vi "FPGA Main (3 Motor).vi"() -> ()   [LabVIEW 2013]
uses:
  Sub VIs/Utilities/Start Boolean.ctl
  <vilib>/Platform/TimedLoop/XDataNode/timing_clust.ctl
  <vilib>/Platform/TimedLoop/XDataNode/nitl_modes.ctl
  <vilib>/Platform/TimedLoop/XDataNode/wakeup.ctl
  <vilib>/rvi/Emulation/niFpgaSctlEmulationGetInTimedLoop.vi
  <vilib>/rvi/Emulation/niFpgaEmulationReportErrorSimple.vi
  <vilib>/rvi/Emulation/niFpgaGetClockAttributes.vi
  <vilib>/rvi/Emulation/niFpgaCriticalErrorInLSC.vi
  <vilib>/rvi/eio/common/nirviEmuTemplateMethod_errors.vi
  <vilib>/rvi/eio/common/nirviEmuTemplatePropertyGet_noerrors.vi
  <vilib>/rvi/interface/RandomDataEmulation/nirviRandomDataFPGAFIFO.vi
  <vilib>/rvi/interface/RandomDataEmulation/niFpgaRandomDataHandleErrors.vi
  <vilib>/Platform/TimedLoop/XDataNode/XDataNode.xnode
  <vilib>/eio/EIONode/EIONode.xnode
  <vilib>/eio/EIOPropertyNode/EIOPropertyNode.xnode
  <vilib>/rvi/DataTransferAndStorage/Container/XNode/niFpgaContainer.xnode
  <vilib>/rvi/interface/RandomDataEmulation/nirviRandomDataFpgaReadWriteTemplate.vi
  <vilib>/Platform/TimedLoop/XDataNode/XDNodeRunTimeDep.lvlib
  <vilib>/rvi/eio/common/nirviEmuTemplatePropertyGet_errors.vi
  <vilib>/rvi/eio/common/nirviEmuTemplatePropertySet_errors.vi
  <vilib>/rvi/eio/common/nirviEmuTemplatePropertySet_noerrors.vi
panel:
  out "Diff_EncC0":u32
  out "Diff_EncB":u32
  out "Diff_EncA":u32
  in  "ABS Enc Channel":u8=255
  in  "Recieved (ticks)":u32=1389
  out "SYS.ACC_SCALE.RDY":bool
  out "ACC.SCALE.WGHT":u16
  out "AO.A_0.WGHT":u32
  out "AO.A_1.WGHT":u32
  out "AO.C_0.WGHT":u32
  out "AO.C_1.WGHT":u32
  out "AO.AudioOut_L.WGHT":u32
  out "AO.AudioOut_R.WGHT":u32
  out "AO.A_0.OFST":u32
  out "AO.C_0.OFST":u32
  out "AO.C_1.OFST":u32
  out "AO.AudioOut_L.OFST":u32
  out "AO.AudioOut_R.OFST":u32
  out "AO.A_1.OFST":u32
  out "SYS.AO_SCALE.RDY":bool
  out "AO.B_0.WGHT":u32
  out "AO.B_1.WGHT":u32
  out "AO.B_0.OFST":u32
  out "AO.B_1.OFST":u32
  out "AI.A_0.WGHT":u32
  out "AI.A_1.WGHT":u32
  out "AI.A_2.WGHT":u32
  out "AI.A_3.WGHT":u32
  out "AI.B_0.WGHT":u32
  out "AI.B_2.WGHT":u32
  out "AI.B_3.WGHT":u32
  out "AI.C_0.WGHT":u32
  out "AI.C_1.WGHT":u32
  out "AI.AudioIn_L.WGHT":u32
  out "AI.AudioIn_R.WGHT":u32
  out "AI.A_0.OFST":u32
  out "AI.A_2.OFST":u32
  out "AI.A_3.OFST":u32
  out "AI.B_0.OFST":u32
  out "AI.B_1.OFST":u32
  out "AI.B_2.OFST":u32
  out "AI.B_3.OFST":u32
  out "AI.C_0.OFST":u32
  out "AI.C_1.OFST":u32
  out "AI.AudioIn_L.OFST":u32
  out "AI.AudioIn_R.OFST":u32
  out "AI.A_1.OFST":u32
  out "SYS.AI_SCALE.RDY":bool
  out "AI.B_1.WGHT":u32
  out "ACC.Z.VAL":u16
  out "SYS.ACC.RDY":bool
  out "ACC.Y.VAL":u16
  out "ACC.X.VAL":u16
  in  "DO.LED3:0":u8 format="%04b"
  out "DI.BTN":u8 format="%08b"
  in  "SYS.SELECTB":u8 format="%08b"
  in  "DIO.B_7:0.DIR":u8 format="%08b"
  in  "DIO.B_7:0.OUT":u8 format="%08b"
  in  "DIO.B_15:8.DIR":u8 format="%08b"
  in  "DIO.B_15:8.OUT":u8 format="%08b"
  out "DIO.B_7:0.IN":u8 format="%08b"
  out "DIO.B_15:8.IN":u8 format="%08b"
  in  "ENC.B.CNFG":u8 format="%08b"
  out "ENC.B.CNTR":u32
  out "ENC.B.STAT":u8 format="%08b"
  out "SYS.RDY":bool
  out "AI.A_0.VAL":u16
  out "AI.A_1.VAL":u16
  out "AI.A_2.VAL":u16
  out "AI.A_3.VAL":u16
  out "AI.B_0.VAL":u16
  out "AI.B_1.VAL":u16
  out "AI.B_2.VAL":u16
  out "AI.B_3.VAL":u16
  out "SYS.AI.RDY":bool
  out "AI.AudioIn_L.VAL":u16
  out "AI.AudioIn_R.VAL":u16
  out "AI.C_1.VAL":u16
  out "AI.C_0.VAL":u16
  in  "AO.A_0.VAL":u16
  in  "AO.A_1.VAL":u16
  in  "AO.B_0.VAL":u16
  in  "AO.B_1.VAL":u16
  in  "AO.AudioOut_L.VAL":u16
  in  "AO.AudioOut_R.VAL":u16
  in  "AO.SYS.GO":T1
  in  "AO.C_1.VAL":u16
  in  "AO.C_0.VAL":u16
  out "AO.SYS.STAT":bool
  in  "SYS.SELECTA":u8 format="%08b"
  in  "DIO.A_7:0.OUT":u8 format="%08b"
  in  "DIO.A_7:0.DIR":u8 format="%08b"
  out "DIO.A_7:0.IN":u8 format="%08b"
  in  "DIO.A_15:8.OUT":u8 format="%08b"
  in  "DIO.A_15:8.DIR":u8 format="%08b"
  out "DIO.A_15:8.IN":u8 format="%08b"
  in  "PWM.A_0.MAX":u16
  in  "PWM.A_0.CMP":u16
  in  "PWM.A_0.CNFG":u8 format="%08b"
  in  "PWM.A_0.CS":u8
  out "PWM.A_0.CNTR":u16
  in  "PWM.A_1.CMP":u16
  in  "PWM.A_1.MAX":u16
  out "PWM.A_1.CNTR":u16
  in  "PWM.A_1.CNFG":u8 format="%08b"
  in  "PWM.A_1.CS":u8
  in  "PWM.A_2.CMP":u16
  in  "PWM.A_2.MAX":u16
  out "PWM.A_2.CNTR":u16
  in  "PWM.A_2.CNFG":u8 format="%08b"
  in  "PWM.A_2.CS":u8
  in  "ENC.A.CNFG":u8 format="%08b"
  out "ENC.A.CNTR":u32
  out "ENC.A.STAT":u8 format="%08b"
  out "DIO.C_7:0.IN":u8 format="%08b"
  in  "DIO.C_7:0.DIR":u8 format="%08b"
  in  "DIO.C_7:0.OUT":u8 format="%08b"
  in  "ENC.C_0.CNFG":u8 format="%08b"
  out "ENC.C_0.CNTR":u32
  out "ENC.C_0.STAT":u8 format="%08b"
  in  "SYS.SELECTC":u8 format="%08b"
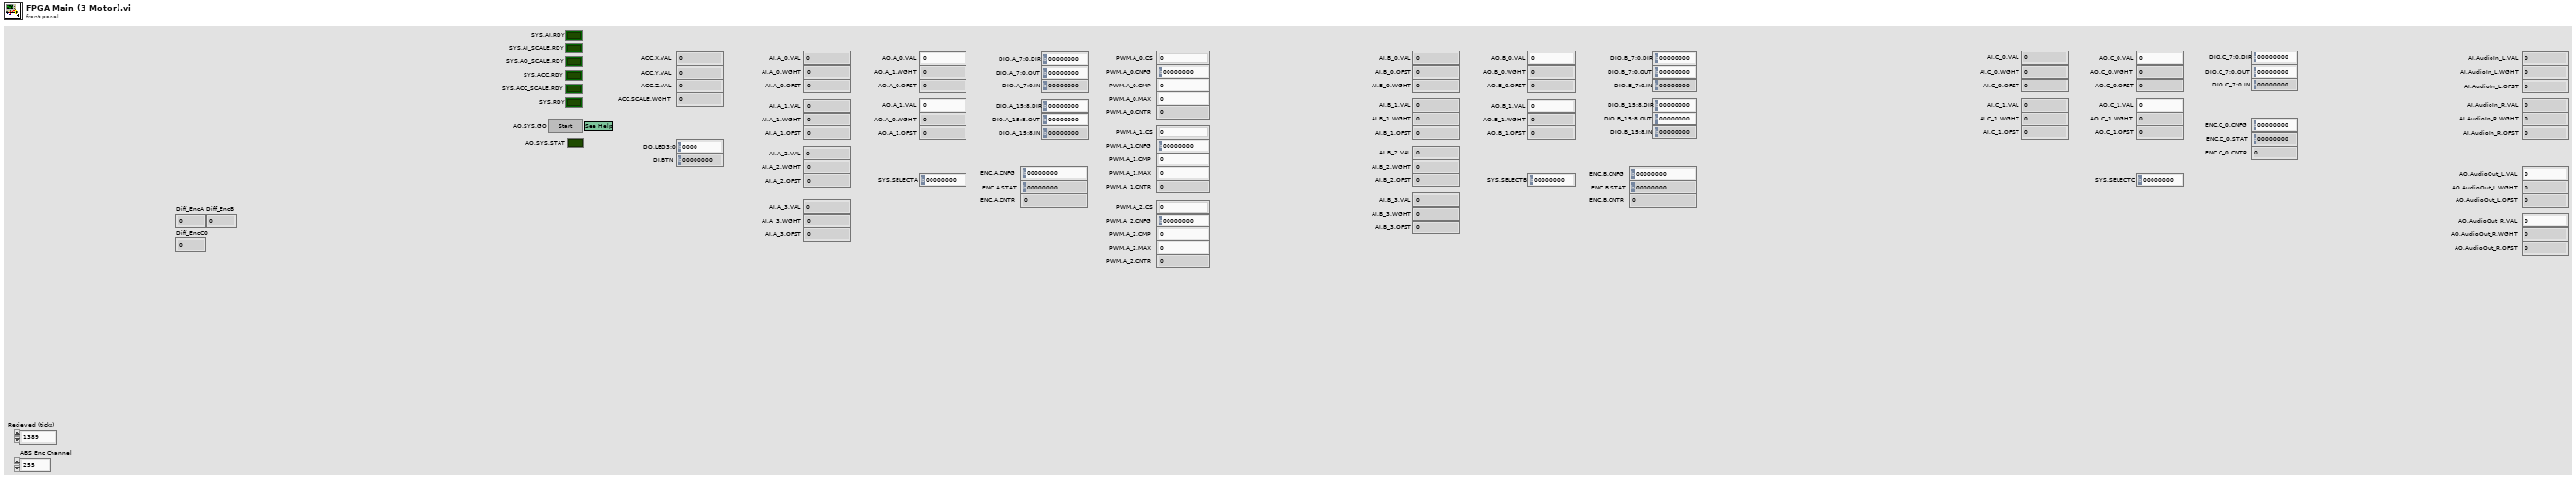
[diagram p1: front panel]
types:
  T1 = typedef "Start Boolean.ctl" = bool
  T2 = typedef "XDNodeRunTimeDep.lvlib/timing_clust.ctl" = cluster{"Expected End [f-1]":u64, "Actual End [f-1]":u64, "Finished Late? [f-1]":bool, "Expected End [i-1]":u64, "Actual End [i-1]":u64, "Finished Late? [i-1]":bool, "Expected Start [i]":u64, "Actual Start [i]":u64, "Expected Start [f]":u64, "Actual Start [f]":u64, "Source Name":string, "Structure Name":string, "Period":i64, "Deadline":i64, "Offset":i64, "Start":i64, "Priority":i32, "Timeout":i32, "Mode":T3, "Wakeup Reason":T4, "Error":errorcluster, "Source Type":string, "Secondary Source Type":string, "Global End Time":u64, "Global Start Time":u64, "Frame Duration":u64, "Iteration Duration":u64, "Assigned CPU":i32, "I/O Scan Engine Mode":u32}
  T3 = typedef "XDNodeRunTimeDep.lvlib/nitl_modes.ctl" = enum32{"No Change", "Process missed periods, maintain original phase", "Discard missed periods, maintain original phase", "Process missed periods, ignore original phase", "Discard missed periods, ignore original phase"}
  T4 = typedef "XDNodeRunTimeDep.lvlib/wakeup.ctl" = enum32{"Normal", "Aborted", "Asynchronous wakeup", "Timing source error", "Timed loop error", "Timeout"}
diagram:
  w1 = u32 0 ("ENC.B.CNTR")
  # "NOTE: The SYS.RDY boolean MUST exist and must become TRUE at some point otherwise the myRIO API will not function correctly."
  # "All DIO operations occur inside one single cycle timed loop (SCTL) since the IO is shared."
  # "The analog input scaling values are stored on the hardware. The RDY boolean should be checked before the values are used otherwise the analog input vlaues could be scaled incorrectly.\n\nAfter the first iteration of the while loop, all indicators have valid values."
  # "The analog output scaling values are stored on the hardware. The RDY boolean should be checked before the values are used otherwise the analog output vlaues could be scaled incorrectly.\n\nAfter the first iteration of the while loop, all indicators have valid values."
  # "The accelerometer nodes takes some time before the values can first be read (this is due to the time taken to read from the acceleromter). An iteration of the while loop will not complete until the accelerometer values have been read.\n\nAfter the first iteration of the while loop, all indicators have valid values."
  # "The onboard accelerometer has a range of +/- 8g which translates to 256 bits/g. The scaling weight is hardcoded in the FPGA to allow for future updates with minimal changes in the myRIO code. The RDY boolean should be checked before the values are used otherwise the analog output vlaues could be scaled incorrectly.\n\nAfter the first iteration of the while loop, all indicators have valid values."
  # "Onboard Accelerometer Scaling"
  # "Analog Output Scaling Constants"
  # "Analog Input Scaling Constants"
  # "Onboard Accelerometer"
  # "Onboard DIO"
  # "Connector B DIO"
  # "There is some delay between when the FPGA code starts and the analog inputs, accelerometer, and scaling values outputs are valid. If the host wants to ensure that there are valid values in theses registers it should wait for each subsystem to finish its initialization process. \n\nWhen all subsystems have finished initializinig, the SYS.RDY indicator will be true, which can be polled by the host to determine the status of the FPGA. Alternatively, the host can poll the individual SYS.xx.RDY indicators to determine the status of the individual subsystems.\n\nThis loop continues indefinitely, essentially making SYS.RDY a read-only register."
  # "The analog input nodes takes some time before the values can first be read (this is due to the time taken to setup the ADC and convert the first reading). An iteration of the while loop will not complete until all the analog input channels have been sampled.\n\nAfter the first iteration of the while loop, all indicators have valid values."
  # "Note: On some hardware a \"ghosting effect\" may occur on any unconnected AI channels. For example, if channel AI0 is connected and channels AI1 - AI7 are not connected the the value read at AI0 may be seen on indicators AI1 - AI7. This is common for hardware that use a multiplexed (MUXed) Analog-to-Digital converter (ADC) since the input analog signal is used to charge a capacitor which does not discharge before the unconnected channel is read.\n\n\"Ghosting\" effect can be hidden be using an mask register which will be used to decide when the indicator should be updated."
  # "The analog output nodes take some time before values are written to the pins. The GO and STAT registers are used to handshake between the FPGA and host. When the host wants the values to be written it sets the GO register to true. If the host reads the STAT register before setting GO, it can then wait for the STAT register value to invert which will tell the host that the output values have been written."
  # "Connector A DIO"
  # "Connector C  DIO"
  # "Host Synchronization"
  # "Analog Output"
  # "Analog Input"
  n1 = while {
    stop <- FALSE stop-if-true
    n2 = local read "SYS.ACC_SCALE.RDY"() -> (w12:bool)
    n3 = local read "SYS.AO_SCALE.RDY"() -> (w13:bool)
    n4 = local read "SYS.AI_SCALE.RDY"() -> (w14:bool)
    n5 = local read "SYS.ACC.RDY"() -> (w15:bool)
    n6 = local read "SYS.AI.RDY"() -> (w17:bool)
    n7 = Compound Arithmetic op=AND(w17, w15, w14, w13, w12) -> (→"SYS.RDY":bool)
  }
  n8 = while {
    i -> [w29]
    stop <- FALSE stop-if-true
    n9 = xnode "FPGA I/O Node"() -> ("ConnectorA/AI0"=→"AI.A_0.VAL":u16, "ConnectorA/AI1"=→"AI.A_1.VAL":u16, "ConnectorA/AI2"=→"AI.A_2.VAL":u16, "ConnectorA/AI3"=→"AI.A_3.VAL":u16, "ConnectorB/AI0"=→"AI.B_0.VAL":u16, "ConnectorB/AI1"=→"AI.B_1.VAL":u16, "ConnectorB/AI2"=→"AI.B_2.VAL":u16, "ConnectorB/AI3"=→"AI.B_3.VAL":u16, "ConnectorC/AI0"=w23:i16, "ConnectorC/AI1"=w22:i16, "AudioIn/Left"=w21:i16, "AudioIn/Right"=w20:i16)  [unwired: 12 in, 12 out]
    n10 = Greater Than 0?(x=w29) -> (x > 0?=→"SYS.AI.RDY":bool)
    n11 = To Unsigned Word Integer(number=w23) -> (unsigned 16bit integer=→"AI.C_0.VAL":u16)
    n12 = To Unsigned Word Integer(number=w22) -> (unsigned 16bit integer=→"AI.C_1.VAL":u16)
    n13 = To Unsigned Word Integer(number=w21) -> (unsigned 16bit integer=→"AI.AudioIn_L.VAL":u16)
    n14 = To Unsigned Word Integer(number=w20) -> (unsigned 16bit integer=→"AI.AudioIn_R.VAL":u16)
  }
  n15 = while {
    i -> [w39]
    stop <- FALSE stop-if-true
    n16 = Greater Than 0?(x=w39) -> (x > 0?=→"SYS.AI_SCALE.RDY":bool)
    n17 = xnode "FPGA I/O Property Node"("FPGA I/O In"=refnum<k21> "ConnectorA/AI0" ("FPGA I/O")) -> ("LSB Weight"=→"AI.A_0.WGHT":u32, "Offset"=w64:i32)  [unwired: 1 out]
    n18 = xnode "FPGA I/O Property Node"("FPGA I/O In"=refnum<k21> "ConnectorA/AI1" ("FPGA I/O")) -> ("LSB Weight"=→"AI.A_1.WGHT":u32, "Offset"=w52:i32)  [unwired: 1 out]
    n19 = xnode "FPGA I/O Property Node"("FPGA I/O In"=refnum<k21> "ConnectorA/AI2" ("FPGA I/O")) -> ("LSB Weight"=→"AI.A_2.WGHT":u32, "Offset"=w61:i32)  [unwired: 1 out]
    n20 = xnode "FPGA I/O Property Node"("FPGA I/O In"=refnum<k21> "ConnectorA/AI3" ("FPGA I/O")) -> ("LSB Weight"=→"AI.A_3.WGHT":u32, "Offset"=w60:i32)  [unwired: 1 out]
    n21 = xnode "FPGA I/O Property Node"("FPGA I/O In"=refnum<k21> "ConnectorB/AI0" ("FPGA I/O")) -> ("LSB Weight"=→"AI.B_0.WGHT":u32, "Offset"=w59:i32)  [unwired: 1 out]
    n22 = xnode "FPGA I/O Property Node"("FPGA I/O In"=refnum<k21> "ConnectorB/AI1" ("FPGA I/O")) -> ("LSB Weight"=→"AI.B_1.WGHT":u32, "Offset"=w58:i32)  [unwired: 1 out]
    n23 = xnode "FPGA I/O Property Node"("FPGA I/O In"=refnum<k21> "ConnectorB/AI2" ("FPGA I/O")) -> ("LSB Weight"=→"AI.B_2.WGHT":u32, "Offset"=w57:i32)  [unwired: 1 out]
    n24 = xnode "FPGA I/O Property Node"("FPGA I/O In"=refnum<k21> "ConnectorB/AI3" ("FPGA I/O")) -> ("LSB Weight"=→"AI.B_3.WGHT":u32, "Offset"=w56:i32)  [unwired: 1 out]
    n25 = xnode "FPGA I/O Property Node"("FPGA I/O In"=refnum<k21> "ConnectorC/AI0" ("FPGA I/O")) -> ("LSB Weight"=→"AI.C_0.WGHT":u32, "Offset"=w55:i32)  [unwired: 1 out]
    n26 = xnode "FPGA I/O Property Node"("FPGA I/O In"=refnum<k21> "ConnectorC/AI1" ("FPGA I/O")) -> ("LSB Weight"=→"AI.C_1.WGHT":u32, "Offset"=w54:i32)  [unwired: 1 out]
    n27 = xnode "FPGA I/O Property Node"("FPGA I/O In"=refnum<k21> "AudioIn/Left" ("FPGA I/O")) -> ("LSB Weight"=→"AI.AudioIn_L.WGHT":u32, "Offset"=w53:i32)  [unwired: 1 out]
    n28 = xnode "FPGA I/O Property Node"("FPGA I/O In"=refnum<k21> "AudioIn/Right" ("FPGA I/O")) -> ("LSB Weight"=→"AI.AudioIn_R.WGHT":u32, "Offset"=w63:i32)  [unwired: 1 out]
    n29 = To Unsigned Long Integer(number=w64) -> (unsigned 32bit integer=→"AI.A_0.OFST":u32)
    n30 = To Unsigned Long Integer(number=w52) -> (unsigned 32bit integer=→"AI.A_1.OFST":u32)
    n31 = To Unsigned Long Integer(number=w61) -> (unsigned 32bit integer=→"AI.A_2.OFST":u32)
    n32 = To Unsigned Long Integer(number=w60) -> (unsigned 32bit integer=→"AI.A_3.OFST":u32)
    n33 = To Unsigned Long Integer(number=w59) -> (unsigned 32bit integer=→"AI.B_0.OFST":u32)
    n34 = To Unsigned Long Integer(number=w58) -> (unsigned 32bit integer=→"AI.B_1.OFST":u32)
    n35 = To Unsigned Long Integer(number=w57) -> (unsigned 32bit integer=→"AI.B_2.OFST":u32)
    n36 = To Unsigned Long Integer(number=w56) -> (unsigned 32bit integer=→"AI.B_3.OFST":u32)
    n37 = To Unsigned Long Integer(number=w55) -> (unsigned 32bit integer=→"AI.C_0.OFST":u32)
    n38 = To Unsigned Long Integer(number=w54) -> (unsigned 32bit integer=→"AI.C_1.OFST":u32)
    n39 = To Unsigned Long Integer(number=w53) -> (unsigned 32bit integer=→"AI.AudioIn_L.OFST":u32)
    n40 = To Unsigned Long Integer(number=w63) -> (unsigned 32bit integer=→"AI.AudioIn_R.OFST":u32)
  }
  n41 = while {
    stop <- FALSE stop-if-true
    n42 = feedback #1(FALSE) -> (w90:bool)
    n43 = case shown="True" "AO.SYS.GO" {
      tunnel: "AO.C_0.VAL" -> [_ w112]
      tunnel: "AO.C_1.VAL" -> [_ w111]
      tunnel: "AO.A_0.VAL" -> [_ w116]
      tunnel: "AO.A_1.VAL" -> [_ w115]
      tunnel: "AO.B_0.VAL" -> [_ w114]
      tunnel: "AO.B_1.VAL" -> [_ w113]
      tunnel: "AO.AudioOut_L.VAL" -> [_ w108]
      tunnel: "AO.AudioOut_R.VAL" -> [_ w107]
      tunnel: w90 -> [w101 w104]
      tunnel: [w101 w102] -> w88
      frame False {
      }
      frame True {
        n44 = To Word Integer(number=w112) -> (16bit integer=w110:i16)
        n45 = To Word Integer(number=w111) -> (16bit integer=w109:i16)
        n46 = To Word Integer(number=w108) -> (16bit integer=w106:i16)
        n47 = To Word Integer(number=w107) -> (16bit integer=w105:i16)
        n48 = flat-sequence {
          tunnel: w116 -> [w125]
          tunnel: w115 -> [w124]
          tunnel: w114 -> [w123]
          tunnel: w113 -> [w122]
          tunnel: w110 -> [w121]
          tunnel: w109 -> [w120]
          tunnel: w106 -> [w119]
          tunnel: w105 -> [w118]
          tunnel: w104 -> [w117]
          tunnel: [w117] -> w103
          tunnel: w103 -> [w127]
          tunnel: [w126] -> w102
          frame #0 {
            n49 = xnode "FPGA I/O Node"("ConnectorA/AO0"=w125, "ConnectorA/AO1"=w124, "ConnectorB/AO0"=w123, "ConnectorB/AO1"=w122, "ConnectorC/AO0"=w121, "ConnectorC/AO1"=w120, "AudioOut/Left"=w119, "AudioOut/Right"=w118) -> ()  [unwired: 8 in, 8 out]
          }
          frame #1 {
            n50 = Not(x=w127) -> (.not. x?=w126:bool)
          }
        }
      }
    }
    "AO.SYS.STAT" <- w88
    n51 = feedback-in #1(w88) -> ()
  }
  n52 = while {
    i -> [w149]
    stop <- FALSE stop-if-true
    n53 = Greater Than 0?(x=w149) -> (x > 0?=→"SYS.AO_SCALE.RDY":bool)
    n54 = xnode "FPGA I/O Property Node"("FPGA I/O In"=refnum<k21> "ConnectorA/AO0" ("FPGA I/O")) -> ("LSB Weight"=→"AO.A_0.WGHT":u32, "Offset"=w160:i32)  [unwired: 1 out]
    n55 = xnode "FPGA I/O Property Node"("FPGA I/O In"=refnum<k21> "ConnectorA/AO1" ("FPGA I/O")) -> ("LSB Weight"=→"AO.A_1.WGHT":u32, "Offset"=w152:i32)  [unwired: 1 out]
    n56 = xnode "FPGA I/O Property Node"("FPGA I/O In"=refnum<k21> "ConnectorB/AO0" ("FPGA I/O")) -> ("LSB Weight"=→"AO.B_0.WGHT":u32, "Offset"=w158:i32)  [unwired: 1 out]
    n57 = xnode "FPGA I/O Property Node"("FPGA I/O In"=refnum<k21> "ConnectorB/AO1" ("FPGA I/O")) -> ("LSB Weight"=→"AO.B_1.WGHT":u32, "Offset"=w157:i32)  [unwired: 1 out]
    n58 = xnode "FPGA I/O Property Node"("FPGA I/O In"=refnum<k21> "ConnectorC/AO0" ("FPGA I/O")) -> ("LSB Weight"=→"AO.C_0.WGHT":u32, "Offset"=w156:i32)  [unwired: 1 out]
    n59 = xnode "FPGA I/O Property Node"("FPGA I/O In"=refnum<k21> "ConnectorC/AO1" ("FPGA I/O")) -> ("LSB Weight"=→"AO.C_1.WGHT":u32, "Offset"=w155:i32)  [unwired: 1 out]
    n60 = xnode "FPGA I/O Property Node"("FPGA I/O In"=refnum<k21> "AudioOut/Left" ("FPGA I/O")) -> ("LSB Weight"=→"AO.AudioOut_L.WGHT":u32, "Offset"=w154:i32)  [unwired: 1 out]
    n61 = xnode "FPGA I/O Property Node"("FPGA I/O In"=refnum<k21> "AudioOut/Right" ("FPGA I/O")) -> ("LSB Weight"=→"AO.AudioOut_R.WGHT":u32, "Offset"=w153:i32)  [unwired: 1 out]
    n62 = To Unsigned Long Integer(number=w160) -> (unsigned 32bit integer=→"AO.A_0.OFST":u32)
    n63 = To Unsigned Long Integer(number=w152) -> (unsigned 32bit integer=→"AO.A_1.OFST":u32)
    n64 = To Unsigned Long Integer(number=w158) -> (unsigned 32bit integer=→"AO.B_0.OFST":u32)
    n65 = To Unsigned Long Integer(number=w157) -> (unsigned 32bit integer=→"AO.B_1.OFST":u32)
    n66 = To Unsigned Long Integer(number=w156) -> (unsigned 32bit integer=→"AO.C_0.OFST":u32)
    n67 = To Unsigned Long Integer(number=w155) -> (unsigned 32bit integer=→"AO.C_1.OFST":u32)
    n68 = To Unsigned Long Integer(number=w154) -> (unsigned 32bit integer=→"AO.AudioOut_L.OFST":u32)
    n69 = To Unsigned Long Integer(number=w153) -> (unsigned 32bit integer=→"AO.AudioOut_R.OFST":u32)
  }
  n70 = node-c288() -> (w4:T2)  [unwired: 1 in]
  n71 = timed-loop {
    timing: w4 -> [_]
    timing-out: [_] -> w3
    stop <- _ stop-if-true
    n72 = xnode "FPGA I/O Node"() -> ("Button0"=w171:bool)  [unwired: 1 in, 1 out]
    n73 = Number To Boolean Array(number="DO.LED3:0") -> (Boolean array=w167:bool[])
    n74 = Build Array(w171) -> (w170:bool[])
    n75 = Index Array(array=w167) -> (element #1=w166:bool, element #2=w165:bool, element #3=w164:bool, element #4=w163:bool)  [unwired: 4 in]
    n76 = Boolean Array To Number(Boolean array=w170) -> (number=→"DI.BTN":u8)
    n77 = xnode "FPGA I/O Node"("LED0"=w166, "LED1"=w165, "LED2"=w164, "LED3"=w163) -> ()  [unwired: 4 in, 4 out]
  }
  n78 = while {
    i -> [w178]
    stop <- FALSE stop-if-true
    n79 = xnode "FPGA I/O Node"() -> ("AccelerationX"=w181:i16, "AccelerationY"=w180:i16, "AccelerationZ"=w179:i16)  [unwired: 3 in, 3 out]
    n80 = Greater Than 0?(x=w178) -> (x > 0?=→"SYS.ACC.RDY":bool)
    n81 = To Unsigned Word Integer(number=w181) -> (unsigned 16bit integer=→"ACC.X.VAL":u16)
    n82 = To Unsigned Word Integer(number=w180) -> (unsigned 16bit integer=→"ACC.Y.VAL":u16)
    n83 = To Unsigned Word Integer(number=w179) -> (unsigned 16bit integer=→"ACC.Z.VAL":u16)
  }
  n84 = while {
    i -> [w185]
    stop <- FALSE stop-if-true
    # "The onboard accelerometer has a range of +/-8g which translates to 256 bits / g. The scaling weight is hardcoded in the FPGA to"
    n85 = Greater Than 0?(x=w185) -> (x > 0?=→"SYS.ACC_SCALE.RDY":bool)
    "ACC.SCALE.WGHT" <- u16 256 ("ACC.SCALE.WGHT")
  }
  n86 = node-c288(w3) -> ()
  n87 = node-c288() -> (w8:T2)  [unwired: 1 in]
  n88 = while {
    stop <- FALSE stop-if-true
    n89 = flat-sequence {
      frame #0 {
        n90 = call "Loop Timer"("Count(Ticks)"="Recieved (ticks)") -> ()  [unwired: 1 out]
      }
      frame #1 {
        n91 = Greater Or Equal?(x="ABS Enc Channel", y=u8 3) -> (x >= y?=w190:bool)
        n92 = case shown="False" w190 {
          tunnel: "ABS Enc Channel" -> [w193 _]
          frame False {
            n93 = local read "DIO.A_15:8.IN"() -> (w207:u8)
            n94 = local read "DIO.B_15:8.IN"() -> (w202:u8)
            n95 = local read "DIO.C_7:0.IN"() -> (w199:u8)
            n96 = Number To Boolean Array(number=w207) -> (Boolean array=w206:bool[])
            n97 = Number To Boolean Array(number=w202) -> (Boolean array=w203:bool[])
            n98 = Number To Boolean Array(number=w199) -> (Boolean array=w201:bool[])
            n99 = xnode ("FIFO Method Node")() -> ("Number of Elements to Write"=w211:u32)  [unwired: 1 in, 1 out]
            n100 = Index Array(array=w206, index=3) -> (element=w198:bool)
            n101 = Index Array(array=w203, index=3) -> (element=w197:bool)
            n102 = Index Array(array=w201, index=0) -> (element=w196:bool)
            n103 = Build Array(w198, w197, w196) -> (w195:bool[])
            n104 = Index Array(array=w195, index=w193) -> (element=w194:bool)
            n105 = call "RecieveACmd.vi"("Digit Signal"=w194) -> ("Finished?"=w208:bool, "Cmd"=w212:u8[])  [unwired: 8 in, 1 out]
            n106 = Greater Or Equal?(x=w211, y=u32 8) -> (x >= y?=w209:bool)
            n107 = And(x=w209, y=w208) -> (x .and. y?=w192:bool)
            n108 = case shown="True" w192 {
              tunnel: w212 -> [_ w213]
              frame False {
              }
              frame True {
                n109 = for {
                  tunnel: w213 -> [w215] mode=indexing
                  n110 = xnode ("FIFO Write")("Element"=w215, "Timeout"=i16 0) -> ()  [unwired: 1 in, 2 out]
                }
              }
            }
          }
          frame True {
          }
        }
      }
    }
  }
  n111 = timed-loop {
    timing: w8 -> [_]
    timing-out: [_] -> w7
    stop <- _ stop-if-true
    # "DIO / Encoder"
    # "DIO / I2C Master"
    # "DIO / PWM"
    # "DIO"
    # "DIO"
    n112 = call "Split HDC Bank3 DIO.vi"("IN 7:0"="DIO.A_7:0.DIR") -> ("OUT 3:0"=w229:fxp<+,4,4>, "OUT 7:4"=w228:fxp<+,4,4>)
    n113 = call "Split HDC Bank3 DIO.vi"("IN 7:0"="DIO.A_7:0.OUT") -> ("OUT 3:0"=w232:fxp<+,4,4>, "OUT 7:4"=w231:fxp<+,4,4>)
    n114 = call "Split HDC Function Select.vi"("IN 7:0"="SYS.SELECTA") -> ("OUT 2"=w256:bool, "OUT 3"=w255:bool, "OUT 4"=w254:bool, "OUT 5"=w253:bool)  [unwired: 2 out]
    n115 = call "DIO 4-bit.vi"("DIO0 Refnum"=refnum<k21> "ConnectorA/DIO4" ("DIO Refnum"), "DIO1 Refnum"=refnum<k21> "ConnectorA/DIO5" ("DIO.0/SPI.MISO"), "DIO2 Refnum"=refnum<k21> "ConnectorA/DIO6" ("DIO.1/SPI.MOSI"), "DIR 3:0"=w228, "OUT 3:0"=w231, "DIO3 Refnum"=refnum<k21> "ConnectorA/DIO7" ("DIO.2/SPI.SCLK")) -> ("IN 3:0"=w221:fxp<+,4,4>)  [unwired: 5 in]
    n116 = call "DIO 4-bit.vi"("DIO0 Refnum"=refnum<k21> "ConnectorA/DIO0", "DIO1 Refnum"=refnum<k21> "ConnectorA/DIO1", "DIO2 Refnum"=refnum<k21> "ConnectorA/DIO2", "DIR 3:0"=w229, "OUT 3:0"=w232, "DIO3 Refnum"=refnum<k21> "ConnectorA/DIO3") -> ("IN 3:0"=w222:fxp<+,4,4>)  [unwired: 5 in]
    n117 = call "Join HDC Bank3 DIO.vi"("IN 7:4"=w221, "IN 3:0"=w222) -> ("OUT 7:0"=→"DIO.A_7:0.IN":u8)
    n118 = call "Split HDC Bank2 DIO.vi"("IN 7:0"="DIO.A_15:8.OUT") -> ("OUT 5"=w239:bool, "OUT 7:6"=w218:fxp<+,2,2>, "OUT 4:3"=w241:fxp<+,2,2>, "OUT 2"=w243:bool, "OUT 0"=w247:bool, "OUT 1"=w246:bool)  [unwired: 2 in]
    n119 = call "Split HDC Bank2 DIO.vi"("IN 7:0"="DIO.A_15:8.DIR") -> ("OUT 5"=w238:bool, "OUT 7:6"=w217:fxp<+,2,2>, "OUT 4:3"=w240:fxp<+,2,2>, "OUT 2"=w242:bool, "OUT 0"=w245:bool, "OUT 1"=w244:bool)  [unwired: 2 in]
    n120 = call "DIO_PWM.vi"("DIO.OUT"=w247, "DIO.DIR"=w245, "PWM.CS"="PWM.A_0.CS", "PWM.CNFG"="PWM.A_0.CNFG", "PWM.CMP"="PWM.A_0.CMP", "PWM.MAX"="PWM.A_0.MAX", "DIO/PWM"=refnum<k21> "ConnectorA/DIO8", "SELECT"=w256) -> ("DIO.IN"=w252:bool, "PWM.CNTR"=→"PWM.A_0.CNTR":u16)  [unwired: 10 in]
    n121 = call "DIO_PWM.vi"("DIO.OUT"=w246, "DIO.DIR"=w244, "PWM.CS"="PWM.A_1.CS", "PWM.CNFG"="PWM.A_1.CNFG", "PWM.CMP"="PWM.A_1.CMP", "PWM.MAX"="PWM.A_1.MAX", "DIO/PWM"=refnum<k21> "ConnectorA/DIO9", "SELECT"=w255) -> ("DIO.IN"=w251:bool, "PWM.CNTR"=→"PWM.A_1.CNTR":u16)  [unwired: 10 in]
    n122 = call "DIO_PWM.vi"("DIO.OUT"=w243, "DIO.DIR"=w242, "PWM.CS"="PWM.A_2.CS", "PWM.CNFG"="PWM.A_2.CNFG", "PWM.CMP"="PWM.A_2.CMP", "PWM.MAX"="PWM.A_2.MAX", "DIO/PWM"=refnum<k21> "ConnectorA/DIO10", "SELECT"=w254) -> ("DIO.IN"=w250:bool, "PWM.CNTR"=→"PWM.A_2.CNTR":u16)  [unwired: 10 in]
    n123 = call "DIO_Encoder.vi"("DIO.1:0.OUT"=w241, "DIO.1:0.DIR"=w240, "QE.CNFG"="ENC.A.CNFG", "DIO.1/QE.B"=refnum<k21> "ConnectorA/DIO12", "SELECT"=w253, "DIO.0/QE.A"=refnum<k21> "ConnectorA/DIO11") -> ("DIO.1:0.IN"=w249:fxp<+,2,2>, "QE.CNTR"=→"ENC.A.CNTR":u32, "QE.STAT"=→"ENC.A.STAT":u8)  [unwired: 11 in]
    n124 = call "DIO 1-bit.vi"("DIR"=w238, "OUT"=w239, "DIO Refnum"=refnum<k21> "ConnectorA/DIO13") -> ("IN"=w248:bool)  [unwired: 8 in]
    n125 = call "DIO 2-bit.vi"("DIO0 Refnum"=refnum<k21> "ConnectorA/DIO14" ("DIO.0/I2C.SDA"), "DIR 1:0"=w217, "OUT 1:0"=w218, "DIO1 Refnum"=refnum<k21> "ConnectorA/DIO15" ("DIO.1/I2C.SCL")) -> ("IN 1:0"=w216:fxp<+,2,2>)
    n126 = call "Join HDC Bank2 DIO.vi"("IN 7:6"=w216, "IN 5"=w248, "IN 4:3"=w249, "IN 0"=w252, "IN 2"=w250, "IN 1"=w251) -> ("OUT 7:0"=→"DIO.A_15:8.IN":u8)  [unwired: 4 in]
  }
  n127 = while {
    border: u32 0 ("ENC.A.CNTR") -> [_]
    border: w1 -> [_]
    border: w1 -> [_]
    stop <- FALSE stop-if-true
    n128 = local read "ENC.C_0.CNTR"() -> (w288:u32)
    n129 = local read "ENC.A.CNTR"() -> (w294:u32)
    n130 = local read "ENC.B.CNTR"() -> (w291:u32)
    n131 = feedback #2() -> (w292:u32)
    n132 = feedback-in #2(w291) -> ()
    n133 = feedback-in #3(w294) -> ()
    n134 = feedback #3() -> (w295:u32)
    n135 = feedback #4() -> (w289:u32)
    n136 = feedback-in #4(w288) -> ()
    n137 = call "Loop Timer2"("Count(mSec)"=u8 1) -> ()  [unwired: 1 out]
    n138 = Subtract(x=w291, y=w292) -> (x-y=→"Diff_EncB":u32)
    n139 = Subtract(x=w294, y=w295) -> (x-y=→"Diff_EncA":u32)
    n140 = Subtract(x=w288, y=w289) -> (x-y=→"Diff_EncC0":u32)
  }
  n141 = node-c288(w7) -> ()
  n142 = node-c288() -> (w6:T2)  [unwired: 1 in]
  n143 = timed-loop {
    timing: w6 -> [_]
    timing-out: [_] -> w5
    stop <- _ stop-if-true
    # "DIO / Encoder"
    # "DIO / I2C Master"
    # "DIO / PWM"
    # "DIO"
    # "DIO"
    n144 = call "Split HDC Bank3 DIO.vi"("IN 7:0"="DIO.B_7:0.OUT") -> ("OUT 3:0"=w326:fxp<+,4,4>, "OUT 7:4"=w319:fxp<+,4,4>)
    n145 = call "Split HDC Bank3 DIO.vi"("IN 7:0"="DIO.B_7:0.DIR") -> ("OUT 3:0"=w324:fxp<+,4,4>, "OUT 7:4"=w318:fxp<+,4,4>)
    n146 = call "Split HDC Function Select.vi"("IN 7:0"="SYS.SELECTB") -> ("OUT 5"=w341:bool)  [unwired: 5 out]
    n147 = call "DIO 4-bit.vi"("DIO0 Refnum"=refnum<k21> "ConnectorB/DIO0", "DIO1 Refnum"=refnum<k21> "ConnectorB/DIO1", "DIO2 Refnum"=refnum<k21> "ConnectorB/DIO2", "DIR 3:0"=w324, "OUT 3:0"=w326, "DIO3 Refnum"=refnum<k21> "ConnectorB/DIO3") -> ("IN 3:0"=w317:fxp<+,4,4>)  [unwired: 5 in]
    n148 = call "DIO 4-bit.vi"("DIO0 Refnum"=refnum<k21> "ConnectorB/DIO4" ("DIO Refnum"), "DIO1 Refnum"=refnum<k21> "ConnectorB/DIO5" ("DIO.0/SPI.MISO"), "DIO2 Refnum"=refnum<k21> "ConnectorB/DIO6" ("DIO.1/SPI.MOSI"), "DIR 3:0"=w318, "OUT 3:0"=w319, "DIO3 Refnum"=refnum<k21> "ConnectorB/DIO7" ("DIO.2/SPI.SCLK")) -> ("IN 3:0"=w315:fxp<+,4,4>)  [unwired: 5 in]
    n149 = call "Join HDC Bank3 DIO.vi"("IN 7:4"=w315, "IN 3:0"=w317) -> ("OUT 7:0"=→"DIO.B_7:0.IN":u8)
    n150 = call "Split HDC Bank2 DIO.vi"("IN 7:0"="DIO.B_15:8.OUT") -> ("OUT 5"=w332:bool, "OUT 7:6"=w300:fxp<+,2,2>, "OUT 4:3"=w333:fxp<+,2,2>, "OUT 2"=w305:bool, "OUT 0"=w313:bool, "OUT 1"=w309:bool)  [unwired: 2 in]
    n151 = call "Split HDC Bank2 DIO.vi"("IN 7:0"="DIO.B_15:8.DIR") -> ("OUT 5"=w330:bool, "OUT 7:6"=w299:fxp<+,2,2>, "OUT 4:3"=w331:fxp<+,2,2>, "OUT 2"=w304:bool, "OUT 0"=w312:bool, "OUT 1"=w308:bool)  [unwired: 2 in]
    n152 = call "DIO 1-bit.vi"("DIR"=w312, "OUT"=w313, "DIO Refnum"=refnum<k21> "ConnectorB/DIO8" ("DIO/PWM")) -> ("IN"=w311:bool)  [unwired: 8 in]
    n153 = call "DIO 1-bit.vi"("DIR"=w308, "OUT"=w309, "DIO Refnum"=refnum<k21> "ConnectorB/DIO9" ("DIO/PWM")) -> ("IN"=w307:bool)  [unwired: 8 in]
    n154 = call "DIO 1-bit.vi"("DIR"=w304, "OUT"=w305, "DIO Refnum"=refnum<k21> "ConnectorB/DIO10" ("DIO/PWM")) -> ("IN"=w303:bool)  [unwired: 8 in]
    n155 = call "DIO_Encoder.vi"("DIO.1:0.OUT"=w333, "DIO.1:0.DIR"=w331, "QE.CNFG"="ENC.B.CNFG", "DIO.1/QE.B"=refnum<k21> "ConnectorB/DIO12", "SELECT"=w341, "DIO.0/QE.A"=refnum<k21> "ConnectorB/DIO11") -> ("DIO.1:0.IN"=w329:fxp<+,2,2>, "QE.CNTR"=→"ENC.B.CNTR":u32, "QE.STAT"=→"ENC.B.STAT":u8)  [unwired: 11 in]
    n156 = call "DIO 1-bit.vi"("DIR"=w330, "OUT"=w332, "DIO Refnum"=refnum<k21> "ConnectorB/DIO13") -> ("IN"=w328:bool)  [unwired: 8 in]
    n157 = call "DIO 2-bit.vi"("DIO0 Refnum"=refnum<k21> "ConnectorB/DIO14" ("DIO.0/I2C.SDA"), "DIR 1:0"=w299, "OUT 1:0"=w300, "DIO1 Refnum"=refnum<k21> "ConnectorB/DIO15" ("DIO.1/I2C.SCL")) -> ("IN 1:0"=w298:fxp<+,2,2>)
    n158 = call "Join HDC Bank2 DIO.vi"("IN 7:6"=w298, "IN 5"=w328, "IN 4:3"=w329, "IN 0"=w311, "IN 2"=w303, "IN 1"=w307) -> ("OUT 7:0"=→"DIO.B_15:8.IN":u8)  [unwired: 4 in]
  }
  n159 = node-c288(w5) -> ()
  n160 = node-c288() -> (w10:T2)  [unwired: 1 in]
  n161 = timed-loop {
    timing: w10 -> [_]
    timing-out: [_] -> w9
    stop <- _ stop-if-true
    n162 = call "Split myDAQ DIO.vi"("IN 7:0"="DIO.C_7:0.OUT") -> ("OUT 2, OUT0"=w373:fxp<+,2,2>, "OUT 1"=w372:bool, "OUT 3"=w362:bool, "OUT 7"=w358:bool, "OUT 6, OUT 4"=w353:fxp<+,2,2>, "OUT 5"=w371:bool)  [unwired: 4 in]
    n163 = call "Split myDAQ DIO.vi"("IN 7:0"="DIO.C_7:0.DIR") -> ("OUT 2, OUT0"=w370:fxp<+,2,2>, "OUT 1"=w369:bool, "OUT 3"=w361:bool, "OUT 7"=w357:bool, "OUT 6, OUT 4"=w352:fxp<+,2,2>, "OUT 5"=w368:bool)  [unwired: 4 in]
    n164 = call "Split myDAQ Function Select.vi"("IN 7:0"="SYS.SELECTC") -> ("OUT 0"=w376:bool)  [unwired: 2 in, 3 out]
    n165 = call "DIO 1-bit.vi"("DIR"=w361, "OUT"=w362, "DIO Refnum"=refnum<k21> "ConnectorC/DIO3" ("DIO/PWM")) -> ("IN"=w360:bool)  [unwired: 8 in]
    n166 = call "DIO_Encoder.vi"("DIO.1:0.OUT"=w373, "DIO.1:0.DIR"=w370, "QE.CNFG"="ENC.C_0.CNFG", "DIO.1/QE.B"=refnum<k21> "ConnectorC/DIO2", "SELECT"=w376, "DIO.0/QE.A"=refnum<k21> "ConnectorC/DIO0") -> ("DIO.1:0.IN"=w366:fxp<+,2,2>, "QE.CNTR"=→"ENC.C_0.CNTR":u32, "QE.STAT"=→"ENC.C_0.STAT":u8)  [unwired: 11 in]
    n167 = call "DIO 1-bit.vi"("DIR"=w369, "OUT"=w372, "DIO Refnum"=refnum<k21> "ConnectorC/DIO1") -> ("IN"=w365:bool)  [unwired: 8 in]
    n168 = call "DIO 1-bit.vi"("DIR"=w368, "OUT"=w371, "DIO Refnum"=refnum<k21> "ConnectorC/DIO5") -> ("IN"=w364:bool)  [unwired: 8 in]
    n169 = call "DIO 2-bit.vi"("DIO0 Refnum"=refnum<k21> "ConnectorC/DIO4" ("DIO.0/QE.A"), "DIR 1:0"=w352, "OUT 1:0"=w353, "DIO1 Refnum"=refnum<k21> "ConnectorC/DIO6" ("DIO.1/QE.B")) -> ("IN 1:0"=w351:fxp<+,2,2>)
    n170 = call "DIO 1-bit.vi"("DIR"=w357, "OUT"=w358, "DIO Refnum"=refnum<k21> "ConnectorC/DIO7" ("DIO/PWM")) -> ("IN"=w356:bool)  [unwired: 8 in]
    n171 = call "Join myDAQ DIO.vi"("IN 7"=w356, "IN 5"=w364, "IN 6, IN 4"=w351, "IN 2, IN 0"=w366, "IN 3"=w360, "IN 1"=w365) -> ("IN 7:0"=→"DIO.C_7:0.IN":u8)  [unwired: 4 in]
  }
  n172 = node-c288(w9) -> ()
